vi "Fault Map to List.vi"(11 "Fault map in":T1) -> (3 "List out":string[][](array[string]))   [LabVIEW 2023, in "Fault Monitor.lvlib" / "Fault Monitor.lvclass"]
uses:
  Library/Fault Monitor.lvclass
  Custom Controls/Fault Map.ctl
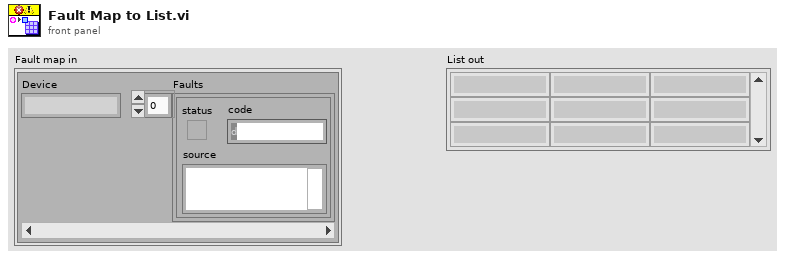
[diagram p1: front panel]
types:
  T1 = typedef "Fault Monitor.lvlib/Fault Monitor.lvclass/Fault Map.ctl" = map{string, errorcluster[]}
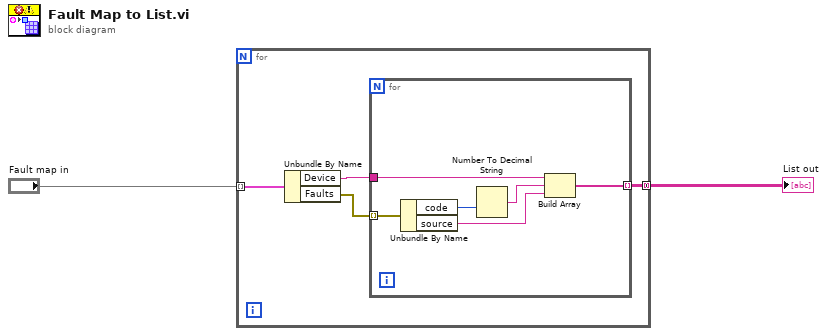
[diagram p0: block diagram]
diagram:
  n1 = for {
    tunnel: "Fault map in" -> [w6] mode=indexing
    tunnel: [w3] -> w2 mode=concatenating
    n2 = Unbundle By Name(w6) -> ("Device"=w4:string, "Faults"=w5:errorcluster[])
    n3 = for {
      tunnel: w5 -> [w11] mode=indexing
      tunnel: w4 -> [w12]
      tunnel: [w7] -> w3 mode=indexing
      n4 = Unbundle By Name(w11) -> ("code"=w10:i32, "source"=w8:string)
      n5 = Number To Decimal String(number=w10) -> (decimal integer string=w9:string)  [unwired: 1 in]
      n6 = Build Array(w12, w9, w8) -> (w7:string[])
    }
  }
  "List out" <- w2
